vi "test Active State.vi"(8 "error in (no error)":errorcluster, 11 "TestCase in":refnum<class "Configuration Tests.lvclass">) -> (0 "error out":errorcluster, 3 "TestCase out":refnum<class "Configuration Tests.lvclass">)   [LabVIEW 2017, in "Configuration Tests.lvclass"]
uses:
  Configuration Tests.lvclass
  <vilib>/addons/_JKI Toolkits/VI Tester/TestCase.llb/TestCase.lvclass
  Classes/Plugin/Plugin.lvclass
  Mock Classes/Plugin/Mock Plugin.lvclass
  Mock Classes/Transfer Group/Mock Transfer Group.lvclass
  Classes/Transfer Group/Transfer Group.lvclass
  C:/github/data-sharing-framework/Data Sharing Framework Core/Engine/Classes/Plugin/Plugin.lvclass
  C:/github/data-sharing-framework/Data Sharing Framework Core/Engine/Classes/Transfer Group/Transfer Group.lvclass
  C:/Program Files (x86)/National Instruments/LabVIEW 2017/vi.lib/addons/_JKI Toolkits/VI Tester/TestCase.llb/TestCase.lvclass
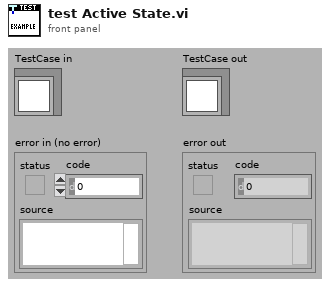
[diagram p1: front panel]
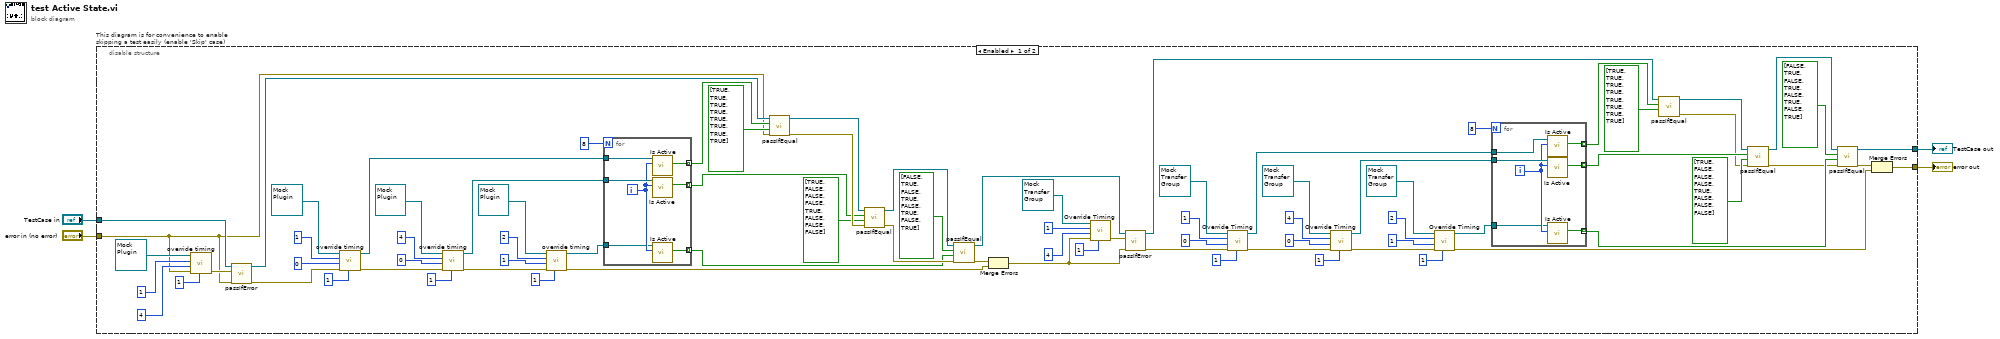
[diagram p0: block diagram]
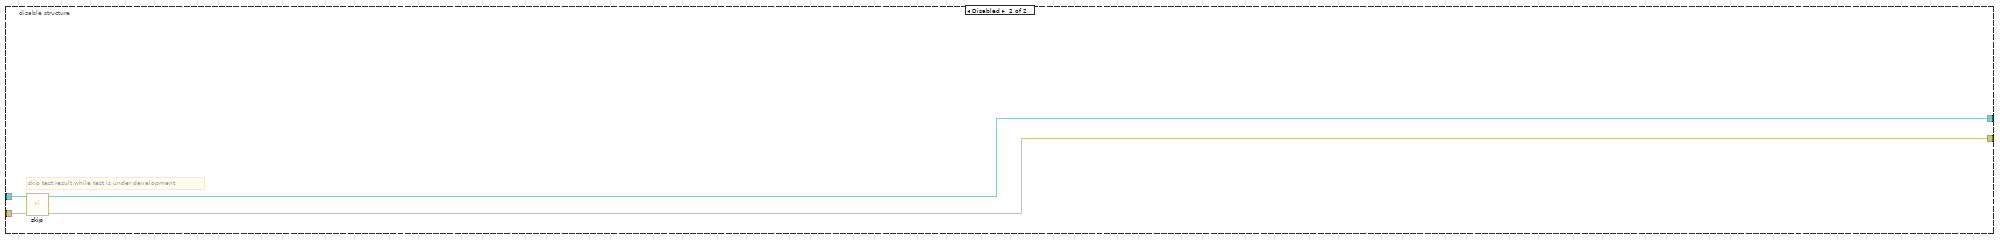
[diagram p2: hidden frame]
diagram:
  n1 = disable-structure "This diagram is for convenience to enable skipping a test easily (enable 'Skip' case)" shown="Enabled" {
    disable-tunnel: "TestCase in" -> [w64 w102]
    disable-tunnel: [w5 w100] -> w1
    disable-tunnel: [w6 w101] -> w3
    disable-tunnel: "error in (no error)" -> [w9 w99]
    frame Enabled {
      n2 = call "override timing.vi"("Priority"=u64 1 ("Offset"), "error in (no error)"=w9, "Offset"=u64 4 ("Priority"), "Decimation"=u64 1, "Mock Plugin in"=refnum<class "Mock Plugin.lvclass"> refnum ("Mock Plugin.lvclass")) -> ("error out"=w62:errorcluster)  [unwired: 5 in, 1 out]
      n3 = call-dynamic "passIfError.vi"("error in (no error)"=w9, "error"=w62, "TestCase in"=w64) -> ("error out"=w60:errorcluster, "TestCase out"=w63:refnum<class "Configuration Tests.lvclass">)  [unwired: 7 in]
      n4 = call "override timing.vi"("Priority"=u64 1 ("Offset"), "error in (no error)"=w60, "Offset"=u64 0 ("Priority"), "Decimation"=u64 1, "Mock Plugin in"=refnum<class "Mock Plugin.lvclass"> refnum ("Mock Plugin.lvclass")) -> ("error out"=w61:errorcluster, "Mock Plugin out"=w83:refnum<class "Mock Plugin.lvclass">)  [unwired: 5 in]
      n5 = call "override timing.vi"("Priority"=u64 1 ("Offset"), "error in (no error)"=w61, "Offset"=u64 0 ("Priority"), "Decimation"=u64 4, "Mock Plugin in"=refnum<class "Mock Plugin.lvclass"> refnum ("Mock Plugin.lvclass")) -> ("error out"=w59:errorcluster, "Mock Plugin out"=w51:refnum<class "Mock Plugin.lvclass">)  [unwired: 5 in]
      n6 = call "override timing.vi"("Priority"=u64 1, "error in (no error)"=w59, "Offset"=u64 1, "Decimation"=u64 2, "Mock Plugin in"=refnum<class "Mock Plugin.lvclass"> refnum) -> ("error out"=w57:errorcluster, "Mock Plugin out"=w49:refnum<class "Mock Plugin.lvclass">)  [unwired: 5 in]
      n7 = for {
        N: 8 -> [_]
        tunnel: w83 -> [w98]
        tunnel: [w97] -> w71 mode=indexing
        tunnel: w51 -> [w96]
        tunnel: [w95] -> w69 mode=indexing
        tunnel: w49 -> [w93]
        tunnel: [w92] -> w47 mode=indexing
        i -> [w94]
        n8 = call "Is Active.vi"("cycle count"=w94, "Plugin in"=w98) -> ("active this cycle?"=w97:bool)  [unwired: 8 in, 1 out]
        n9 = call "Is Active.vi"("cycle count"=w94, "Plugin in"=w96) -> ("active this cycle?"=w95:bool)  [unwired: 8 in, 1 out]
        n10 = call "Is Active.vi"("cycle count"=w94, "Plugin in"=w93) -> ("active this cycle?"=w92:bool)  [unwired: 8 in, 1 out]
      }
      n11 = call-dynamic "passIfEqual.vi"("error in (no error)"=w9, "y"=bool[] [TRUE, TRUE, TRUE, TRUE, TRUE, TRUE, TRUE, TRUE], "x"=w71, "TestCase in"=w63) -> ("error out"=w74:errorcluster, "TestCase out"=w72:refnum<class "Configuration Tests.lvclass">)  [unwired: 6 in]
      n12 = call-dynamic "passIfEqual.vi"("error in (no error)"=w74, "y"=bool[] [TRUE, FALSE, FALSE, FALSE, TRUE, FALSE, FALSE, FALSE], "x"=w69, "TestCase in"=w72) -> ("error out"=w73:errorcluster, "TestCase out"=w52:refnum<class "Configuration Tests.lvclass">)  [unwired: 6 in]
      n13 = call-dynamic "passIfEqual.vi"("error in (no error)"=w73, "y"=w47, "x"=bool[] [FALSE, TRUE, FALSE, TRUE, FALSE, TRUE, FALSE, TRUE], "TestCase in"=w52) -> ("error out"=w53:errorcluster, "TestCase out"=w11:refnum<class "Configuration Tests.lvclass">)  [unwired: 6 in]
      n14 = Merge Errors(w53, w57) -> (w10:errorcluster)
      n15 = call "Override Timing.vi"("Priority"=u64 1 ("Offset"), "error in (no error)"=w10, "Offset"=u64 4 ("Priority"), "Decimation"=u64 1, "Mock Transfer Group in"=refnum<class "Mock Transfer Group.lvclass"> refnum ("Mock Transfer Group.lvclass")) -> ("error out"=w33:errorcluster)  [unwired: 5 in, 1 out]
      n16 = call-dynamic "passIfError.vi"("error in (no error)"=w10, "error"=w33, "TestCase in"=w11) -> ("error out"=w35:errorcluster, "TestCase out"=w32:refnum<class "Configuration Tests.lvclass">)  [unwired: 7 in]
      n17 = call "Override Timing.vi"("Priority"=u64 1 ("Offset"), "error in (no error)"=w35, "Offset"=u64 0 ("Priority"), "Decimation"=u64 1, "Mock Transfer Group in"=refnum<class "Mock Transfer Group.lvclass"> refnum ("Mock Transfer Group.lvclass")) -> ("error out"=w34:errorcluster, "Mock Transfer Group out"=w13:refnum<class "Mock Transfer Group.lvclass">)  [unwired: 5 in]
      n18 = call "Override Timing.vi"("Priority"=u64 1 ("Offset"), "error in (no error)"=w34, "Offset"=u64 0 ("Priority"), "Decimation"=u64 4, "Mock Transfer Group in"=refnum<class "Mock Transfer Group.lvclass"> refnum ("Mock Transfer Group.lvclass")) -> ("error out"=w36:errorcluster, "Mock Transfer Group out"=w42:refnum<class "Mock Transfer Group.lvclass">)  [unwired: 5 in]
      n19 = call "Override Timing.vi"("Priority"=u64 1, "error in (no error)"=w36, "Offset"=u64 1, "Decimation"=u64 2, "Mock Transfer Group in"=refnum<class "Mock Transfer Group.lvclass"> refnum ("Mock Plugin in")) -> ("error out"=w7:errorcluster, "Mock Transfer Group out"=w44:refnum<class "Mock Transfer Group.lvclass">)  [unwired: 5 in]
      n20 = for {
        N: 8 -> [_]
        tunnel: w13 -> [w91]
        tunnel: [w90] -> w25 mode=indexing
        tunnel: w42 -> [w89]
        tunnel: [w88] -> w27 mode=indexing
        tunnel: w44 -> [w86]
        tunnel: [w85] -> w46 mode=indexing
        i -> [w87]
        n21 = call "Is Active.vi"("cycle count"=w87, "Transfer Group in"=w91) -> ("active this cycle?"=w90:bool)  [unwired: 8 in, 1 out]
        n22 = call "Is Active.vi"("cycle count"=w87, "Transfer Group in"=w89) -> ("active this cycle?"=w88:bool)  [unwired: 8 in, 1 out]
        n23 = call "Is Active.vi"("cycle count"=w87, "Transfer Group in"=w86) -> ("active this cycle?"=w85:bool)  [unwired: 8 in, 1 out]
      }
      n24 = call-dynamic "passIfEqual.vi"("y"=bool[] [TRUE, TRUE, TRUE, TRUE, TRUE, TRUE, TRUE, TRUE], "x"=w25, "TestCase in"=w32) -> ("error out"=w22:errorcluster, "TestCase out"=w24:refnum<class "Configuration Tests.lvclass">)  [unwired: 7 in]
      n25 = call-dynamic "passIfEqual.vi"("error in (no error)"=w22, "y"=bool[] [TRUE, FALSE, FALSE, FALSE, TRUE, FALSE, FALSE, FALSE], "x"=w27, "TestCase in"=w24) -> ("error out"=w23:errorcluster, "TestCase out"=w41:refnum<class "Configuration Tests.lvclass">)  [unwired: 6 in]
      n26 = call-dynamic "passIfEqual.vi"("error in (no error)"=w23, "y"=w46, "x"=bool[] [FALSE, TRUE, FALSE, TRUE, FALSE, TRUE, FALSE, TRUE], "TestCase in"=w41) -> ("error out"=w8:errorcluster, "TestCase out"=w5:refnum<class "Configuration Tests.lvclass">)  [unwired: 6 in]
      n27 = Merge Errors(w8, w7) -> (w6:errorcluster)
    }
    frame Disabled {
      # "skip test result while test is under development"
      n28 = call <vilib>:"skip.vi"("error in (no error)"=w99, "TestCase in"=w102) -> ("error out"=w101:errorcluster, "TestCase out"=w100:refnum<class "Configuration Tests.lvclass">)  [unwired: 8 in]
    }
  }
  "error out" <- w3
  "TestCase out" <- w1
